vi "MeasurementServer_GetRequest_Invoke.vi"(6 "error in (no error)":errorcluster, 9 "gRPCid":T1) -> (0 "error out":errorcluster, 1 "parameter":string, 2 "command":string, 3 "gRPCid out":T1)   [LabVIEW 2019, in "labview-grpc-measurement-server.lvlib"]
uses:
  labview-grpc-measurement-server.lvlib
  MeasurementServer_gRPCid.ctl
  MeasurementServer_InvokeRequest.ctl
  home/lvuser/ocv_labview_measurement_server.so
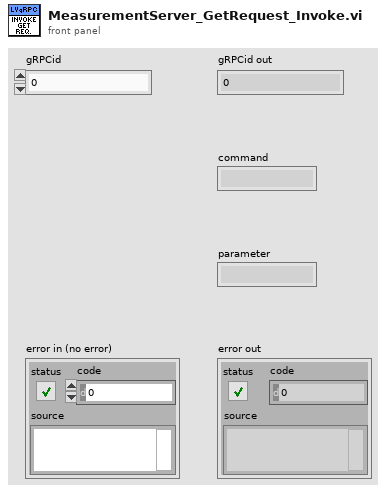
[diagram p1: front panel]
types:
  T1 = typedef "labview-grpc-measurement-server.lvlib/MeasurementServer_gRPCid.ctl" = u64
  T2 = typedef "labview-grpc-measurement-server.lvlib/MeasurementServer_InvokeRequest.ctl" = cluster{"command":string, "parameter":string}
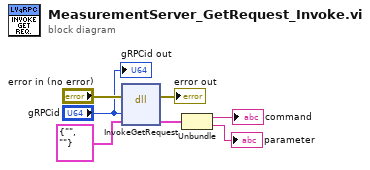
[diagram p0: block diagram]
diagram:
  n1 = dll-call lib="home/lvuser/ocv_labview_measurement_server.so" fn="InvokeGetRequest"(error in="error in (no error)", "id"="gRPCid", "data"=T2 {"command"="", "parameter"=""} ("InvokeRequest")) -> (error out=→"error out":errorcluster, "data"=w3:T2)  [unwired: 4 in, 1 out]
  n2 = Unbundle(w3) -> ("command"=→"command":string, "parameter"=→"parameter":string)
  "gRPCid out" <- "gRPCid"
